vi "纳清蓝绿藻_平均次数写入.vi"(8 "error in (no error)":errorcluster caption="错误输入（无错误）", 10 "数值":u16, 11 "MB session in":refnum<class "MB_Master.lvclass">) -> (0 "error out":errorcluster caption="错误输出", 3 "MB session out":refnum<class "MB_Master.lvclass">)   [LabVIEW 2016, in "斯坦道多参数.lvlib"]
uses:
  <vilib>/Plasmionique/MB Master/MB Master.lvlib
  <vilib>/Plasmionique/MB Master/MB_Master/MB_Master.lvclass
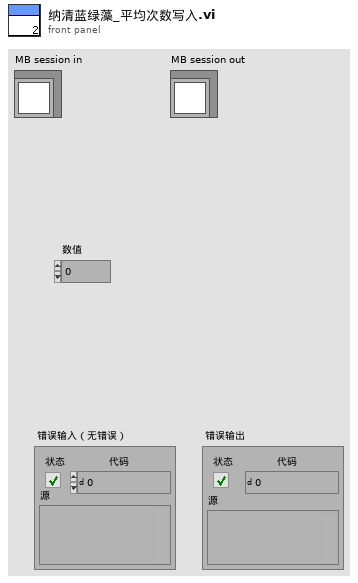
[diagram p1: front panel]
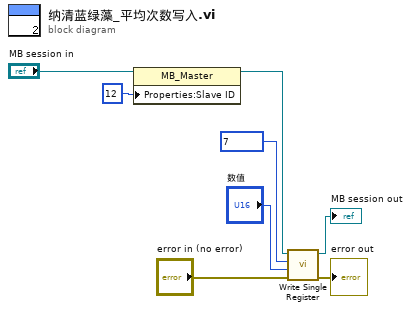
[diagram p0: block diagram]
diagram:
  n1 = property class="MB_Master"(reference="MB session in", "Properties:Slave ID"=u8 12 ("Slave ID")) -> (reference out=w5:refnum<class "MB_Master.lvclass">)  [unwired: 1 in, 1 out]
  n2 = call <vilib>:"Write Single Register.vi"("error in (no error)"="error in (no error)", "value"="数值", "address"=u16 7 ("starting address"), "MB session in"=w5) -> ("error out"=→"error out":errorcluster, "MB session out"=→"MB session out":refnum<class "MB_Master.lvclass">)  [unwired: 6 in]
